vi "FRCts20_Backend_Test_Request.vi"() -> ()   [LabVIEW 2014, in "FRCts20_Backend_TestCode.lvlib"]
uses:
  FRCts20_Backend_TestCode.lvlib
  FRCts20_Backend_Engine.lvlib
  FRCts20_Backend_API/FRCts20_Backend_API_Status.ctl
  FRCts20_Backend_API/FRCts20_Backend_API_Application.vi
  FRCts20_Backend_API/FRCts20_Backend_API_Command_App.ctl
  FRCts20_Backend_API/FRCts20_Backend_API_Request.ctl
panel:
  out "Get Root Pass/Fail":bool
  out "Get ROOT":u32
  out "Get Pass/Fail":bool
  out "error out":errorcluster
  out "Del Pass/Fail":bool
  out "GetDel":u32
  out "Del":u32
  out "GetPut":u32
  out "Put":u32
  out "Put Pass/Fail":bool
  out "Post Pass/Fail":bool
  out "GetPost":u32
  out "post":u32
  out "Get Req 1":u32
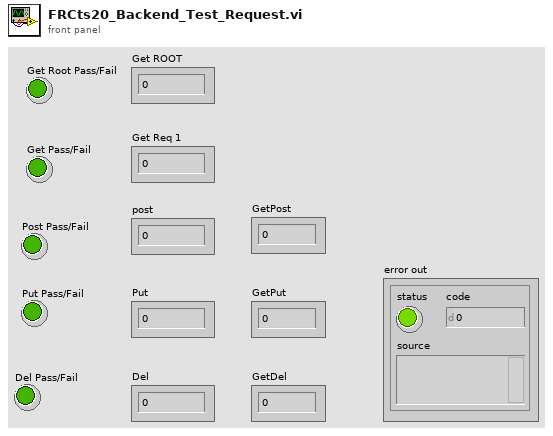
[diagram p1: front panel]
types:
  T1 = typedef "FRCts20_Backend_API.lvlib/FRCts20_Backend_API_Request.ctl" = cluster{"Request Index":u32, "Description":string, "Status":T2, "Open Date":timestamp, "Last Update":timestamp, "Closed Date":timestamp, "Notes":cluster{"Note Index":u32, "Text":string, "Time Entered":timestamp, "Author":string, "Solution":bool}[], "Team Index":u32, "APIReturn":string}
  T2 = typedef "FRCts20_Backend_API.lvlib/FRCts20_Backend_API_Status.ctl" = enum16{"Open", "In Work", "Closed"}
  T3 = typedef "FRCts20_Backend_API.lvlib/FRCts20_Backend_API_Command_App.ctl" = string
  T4 = typedef "FRCts20_Backend_API.lvlib/FRCts20_Backend_API_RequestRoot.ctl" = cluster{"Requests":cluster{"Request Index":u32, "Description":string, "Status":T2, "Open Date":timestamp, "Last Update":timestamp, "Closed Date":timestamp, "Team Index":u32}[], "APIReturn":string}
  T5 = cluster{"Request Index":u32, "Description":string, "Status":T2, "Open Date":timestamp, "Last Update":timestamp, "Closed Date":timestamp, "Team Index":u32}[]
  T6 = cluster{"Request Index":u32, "Description":string, "Status":T2, "Open Date":timestamp, "Last Update":timestamp, "Closed Date":timestamp, "Team Index":u32}
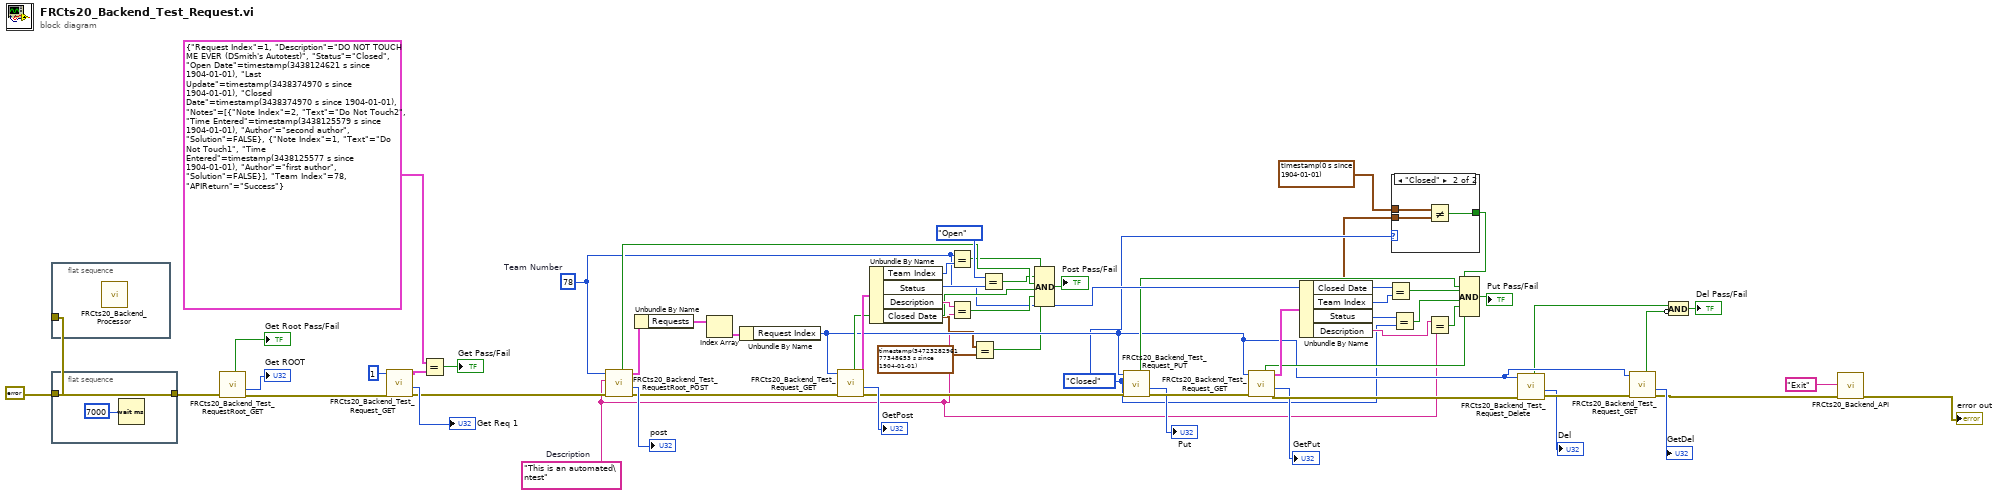
[diagram p0: block diagram]
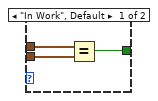
[diagram p2: hidden frame]
diagram:
  w18 = FRCts20_Backend_API_Status."Closed" ("Status In")
  w40 = u32 78  # Team Number
  w6 = "This is an automated\ntest"  # Description
  w62 = errorcluster {"status"=FALSE, "code"=0, "source"=""} ("error constant")
  n1 = flat-sequence {
    tunnel: w62 -> [_]
    frame #0 {
      n2 = call "FRCts20_Backend_Processor.vi"() -> ()  [unwired: 12 in]
    }
  }
  n3 = flat-sequence {
    tunnel: w62 -> [w63]
    tunnel: [w63] -> w5
    frame #0 {
      n4 = Wait (ms)(milliseconds to wait=u32 7000) -> ()  [unwired: 1 out]
    }
  }
  n5 = call "FRCts20_Backend_Test_RequestRoot_GET.vi"("error in (no error)"=w5) -> ("error out"=w4:errorcluster, "Time (ms)"=→"Get ROOT":u32, "Success"=→"Get Root Pass/Fail":bool)  [unwired: 7 in, 1 out]
  n6 = call "FRCts20_Backend_Test_Request_GET.vi"("error in (no error)"=w4, "Request Index"=u32 1) -> ("error out"=w59:errorcluster, "Time (ms)"=→"Get Req 1":u32, "Request Out"=w10:T1)  [unwired: 5 in, 2 out]
  n7 = Equal?(x=T1 {"Request Index"=1, "Description"="DO NOT TOUCH ME EVER (DSmith's Autotest)", "Status"=enum."Closed", "Open Date"=timestamp(3438124621 s since 1904-01-01), "Last Update"=timestamp(3438374970 s since 1904-01-01), "Closed Date"=timestamp(3438374970 s since 1904-01-01), "Notes"=[{"Note Index"=2, "Text"="Do Not Touch2", "Time Entered"=timestamp(3438125579 s since 1904-01-01), "Author"="second author", "Solution"=FALSE}, {"Note Index"=1, "Text"="Do Not Touch1", "Time Entered"=timestamp(3438125577 s since 1904-01-01), "Author"="first author", "Solution"=FALSE}], "Team Index"=78, "APIReturn"="Success"} ("Request Out"), y=w10) -> (x = y?=→"Get Pass/Fail":bool)
  n8 = call "FRCts20_Backend_Test_RequestRoot_POST.vi"("error in (no error)"=w59, "Description"=w6, "Team Index"=w40) -> ("error out"=w57:errorcluster, "Time (ms)"=→"post":u32, "Request Out"=w9:T4, "Success"=w49:bool)  [unwired: 4 in, 1 out]
  n9 = Unbundle By Name(w9) -> ("Requests"=w8:T5)
  n10 = Index Array(array=w8) -> (element=w7:T6)  [unwired: 1 in]
  n11 = Unbundle By Name(w7) -> ("Request Index"=w29:u32)
  n12 = call "FRCts20_Backend_Test_Request_GET.vi"("error in (no error)"=w57, "Request Index"=w29) -> ("error out"=w44:errorcluster, "Time (ms)"=→"GetPost":u32, "Request Out"=w55:T1, "Success"=w50:bool)  [unwired: 5 in, 1 out]
  n13 = Unbundle By Name(w55) -> ("Team Index"=w53:u32, "Status"=w52:T2, "Description"=w54:string, "Closed Date"=w13:timestamp)
  n14 = Equal?(x=w40, y=w53) -> (x = y?=w46:bool)
  n15 = Equal?(x=w54, y=w6) -> (x = y?=w47:bool)
  n16 = Equal?(x=w13, y=timestamp(3.4723282961773486e+18 s since 1904-01-01) ("PutClosedDate")) -> (x = y?=w12:bool)
  n17 = Equal?(x=FRCts20_Backend_API_Status."Open", y=w52) -> (x = y?=w48:bool)
  n18 = Compound Arithmetic op=AND(w46, w48, w49, w50, w47, w12) -> (→"Post Pass/Fail":bool)
  n19 = call "FRCts20_Backend_Test_Request_PUT.vi"("error in (no error)"=w44, "Status In"=w18, "Request Index"=w29) -> ("error out"=w43:errorcluster, "Time (ms)"=→"Put":u32, "Success"=w33:bool)  [unwired: 4 in, 2 out]
  n20 = call "FRCts20_Backend_Test_Request_GET.vi"("error in (no error)"=w43, "Request Index"=w29) -> ("error out"=w31:errorcluster, "Time (ms)"=→"GetPut":u32, "Request Out"=w42:T1, "Success"=w36:bool)  [unwired: 5 in, 1 out]
  n21 = Unbundle By Name(w42) -> ("Closed Date"=w16:timestamp, "Team Index"=w41:u32, "Status"=w39:T2, "Description"=w38:string)
  n22 = Equal?(x=w40, y=w41) -> (x = y?=w34:bool)
  n23 = case shown="\"Closed\"" w18 {
    tunnel: timestamp(0 s since 1904-01-01) ("PutClosedDate") -> [w67 w70]
    tunnel: w16 -> [w66 w69]
    tunnel: [w65 w68] -> w15
    frame "In Work", Default {
      n24 = Equal?(x=w67, y=w66) -> (x = y?=w65:bool)
    }
    frame "Closed" {
      n25 = Not Equal?(x=w70, y=w69) -> (x != y?=w68:bool)
    }
  }
  n26 = Equal?(x=w39, y=w18) -> (x = y?=w35:bool)
  n27 = Equal?(x=w38, y=w6) -> (x = y?=w37:bool)
  n28 = Compound Arithmetic op=AND(w15, w33, w34, w35, w37, w36) -> (→"Put Pass/Fail":bool)
  n29 = call "FRCts20_Backend_Test_Request_Delete.vi"("error in (no error)"=w31, "Request Index"=w29) -> ("error out"=w30:errorcluster, "Time (ms)"=→"Del":u32, "Success"=w23:bool)  [unwired: 5 in, 2 out]
  n30 = call "FRCts20_Backend_Test_Request_GET.vi"("error in (no error)"=w30, "Request Index"=w29) -> ("error out"=w21:errorcluster, "Time (ms)"=→"GetDel":u32, "Success"=w24:bool)  [unwired: 5 in, 2 out]
  n31 = Compound Arithmetic op=AND(w23, invert w24) -> (→"Del Pass/Fail":bool)
  n32 = call-poly "FRCts20_Backend_API.vi"("error in (no error)"=w21, "Command"=T3 "Exit") -> ("error out"=→"error out":errorcluster)  [unwired: 7 in, 2 out]
